vi "OE1022D_Read 1 parameter_mean.vi"(1 "数据转换":u8[](array[numeric]), 5 "Parameter 3":u16(ring) items=["AUX1", "AUX2", "AUX3", "AUX4"], 7 "Parameter 2":u16(ring) items=["X", "Y", "R", "Theta", "Frequency", "Noise", "Xh1", "Yh1", "Rh1", "Theta h1", "Xh2", "Yh2", "Rh2", "Theta h2"], 8 "错误输入（无错误）":errorcluster {"code" format="%f"}, 9 "Parameter":u16(ring) items=["X", "Y", "R", "Theta", "Frequency", "Noise", "Xh1", "Yh1", "Rh1", "Theta h1", "Xh2", "Yh2", "Rh2", "Theta h2"], 10 "Channel (0: A)":u16(ring) items=["Channel A", "Channel B", "ADC"], 11 "VISA resource name":refnum<visa-resource-name>) -> (0 "error out":errorcluster, 2 "Measurement":dbl format="%.3p", 3 "VISA resource name out":refnum<visa-resource-name>)   [LabVIEW 2022 SP3]
uses:
  <vilib>/Analysis/NI_AALBase.lvlib
panel:
  out "Measurement STD":dbl format="%#_13g"
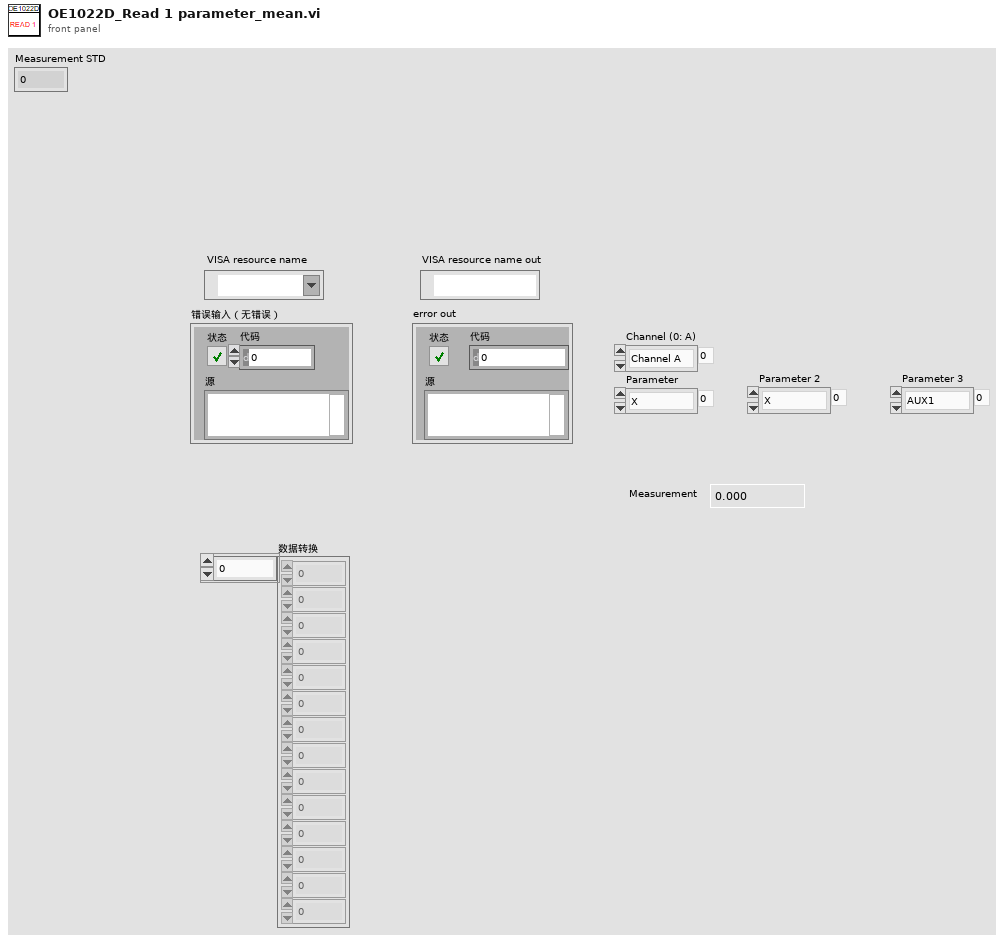
[diagram p1: front panel]
types:
  T1 = cluster{"AD1":dbl[], "AD2":dbl[], "AD3":dbl[], "AD4":dbl[]}
  T2 = cluster{"XA":dbl[], "YA":dbl[], "FrequencyA":dbl[], "NoiseA":dbl[], "Xh1A":dbl[], "Yh1A":dbl[], "Xh2A":dbl[], "Yh2A":dbl[]}
  T3 = cluster{"XB":dbl[], "YB":dbl[], "FrequencyB":dbl[], "NoiseB":dbl[], "Xh1B":dbl[], "Yh1B":dbl[], "Xh2B":dbl[], "Yh2B":dbl[], "Xh2B":dbl[]}
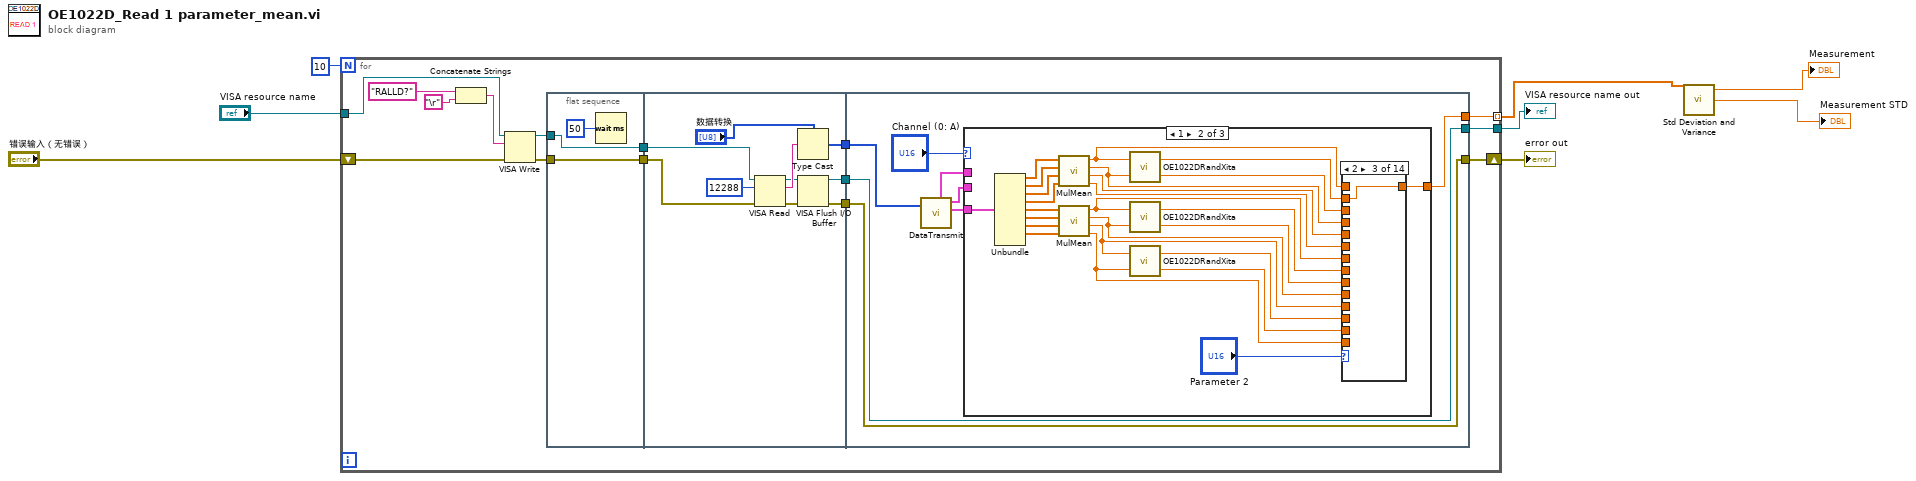
[diagram p0: block diagram]
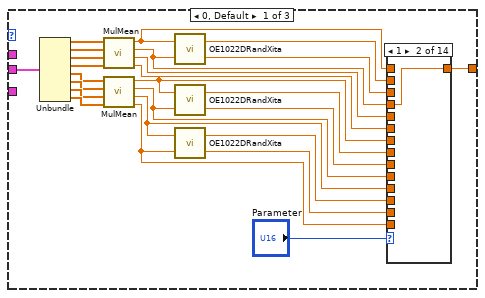
[diagram p2: hidden frame]
diagram:
  n1 = for {
    N: 10 -> [_]
    tunnel: [w13] -> w8
    shift-right: [w12] -> w7
    shift-left: "错误输入（无错误）" -> [w9]
    tunnel: [w11] -> w3 mode=indexing
    tunnel: "VISA resource name" -> [w10]
    n2 = Concatenate Strings("RALLD?" ("命令输入"), "\r") -> (w17:string)
    n3 = VISA Write(VISA resource name=w10, write buffer=w17, error in (no error)=w9) -> (VISA resource name out=w15:refnum<visa-resource-name>, error out=w14:errorcluster)  [unwired: 1 out]
    n4 = flat-sequence {
      tunnel: w15 -> [w24]
      tunnel: w14 -> [w25]
      tunnel: [w25] -> w23
      tunnel: [w24] -> w22
      tunnel: w23 -> [w28]
      tunnel: w22 -> [w27]
      tunnel: [w31] -> w21
      tunnel: [w30] -> w20
      tunnel: [w29] -> w19
      tunnel: w21 -> [w41]
      tunnel: w20 -> [w43]
      tunnel: w19 -> [w42]
      tunnel: [w43] -> w12
      tunnel: [w42] -> w13
      tunnel: [w37] -> w11
      frame #0 {
        n5 = Wait (ms)(milliseconds to wait=u32 50 ("等待时间（毫秒）")) -> ()  [unwired: 1 out]
      }
      frame #1 {
        n6 = VISA Read(VISA resource name=w27, byte count=12288, error in (no error)=w28) -> (VISA resource name out=w33:refnum<visa-resource-name>, read buffer=w35:string, error out=w34:errorcluster)  [unwired: 1 out]
        n7 = Type Cast(type="数据转换", x=w35) -> (*(type *) &x=w31:u8[])
        n8 = VISA Flush I/O Buffer(VISA resource name=w33, error in (no error)=w34) -> (VISA resource name out=w29:refnum<visa-resource-name>, error out=w30:errorcluster)  [unwired: 1 in]
      }
      frame #2 {
        n9 = call "DataTransmit.vi"("数据输入"=w41) -> ("输出簇ADC"=w40:T1, "输出簇A"=w39:T2, "输出簇B"=w38:T3)  [unwired: 2 in, 2 out]
        n10 = case shown="1" "Channel (0: A)" {
          tunnel: w40 -> [_ _ w129]
          tunnel: w39 -> [w60 _ _]
          tunnel: w38 -> [_ w84 _]
          tunnel: [w55 w85 w123] -> w37
          frame 0, Default {
            n11 = Unbundle(w60) -> ("XA"=w61:dbl[], "YA"=w62:dbl[], "FrequencyA"=w63:dbl[], "NoiseA"=w64:dbl[], "Xh1A"=w65:dbl[], "Yh1A"=w66:dbl[], "Xh2A"=w67:dbl[], "Yh2A"=w68:dbl[])
            n12 = call "MulMean.vi"("IN 4"=w64, "IN 3"=w63, "IN 2"=w62, "IN 1"=w61) -> ("mean 4"=w49:dbl, "mean 3"=w50:dbl, "mean 2"=w58:dbl, "mean 1"=w59:dbl)  [unwired: 4 in]
            n13 = call "MulMean.vi"("IN 4"=w68, "IN 3"=w67, "IN 2"=w66, "IN 1"=w65) -> ("mean 4"=w47:dbl, "mean 3"=w48:dbl, "mean 2"=w53:dbl, "mean 1"=w54:dbl)  [unwired: 4 in]
            n14 = call "OE1022DRandXita.vi"("Y"=w58, "X"=w59) -> ("θ (°)"=w56:dbl, "R"=w57:dbl)
            n15 = call "OE1022DRandXita.vi"("Y"=w53, "X"=w54) -> ("θ (°)"=w51:dbl, "R"=w52:dbl)
            n16 = call "OE1022DRandXita.vi"("Y"=w47, "X"=w48) -> ("θ (°)"=w45:dbl, "R"=w46:dbl)
            n17 = case shown="1" "Parameter" {
              tunnel: w59 -> [w70 _ _ _ _ _ _ _ _ _ _ _ _ _]
              tunnel: w58 -> [_ w71 _ _ _ _ _ _ _ _ _ _ _ _]
              tunnel: w57 -> [_ _ w72 _ _ _ _ _ _ _ _ _ _ _]
              tunnel: w56 -> [_ _ _ w73 _ _ _ _ _ _ _ _ _ _]
              tunnel: [w70 w71 w72 w73 w74 w75 w76 w77 w78 w79 w80 w81 w82 w83] -> w55
              tunnel: w54 -> [_ _ _ _ _ _ w76 _ _ _ _ _ _ _]
              tunnel: w53 -> [_ _ _ _ _ _ _ w77 _ _ _ _ _ _]
              tunnel: w52 -> [_ _ _ _ _ _ _ _ w78 _ _ _ _ _]
              tunnel: w51 -> [_ _ _ _ _ _ _ _ _ w79 _ _ _ _]
              tunnel: w50 -> [_ _ _ _ w74 _ _ _ _ _ _ _ _ _]
              tunnel: w49 -> [_ _ _ _ _ w75 _ _ _ _ _ _ _ _]
              tunnel: w48 -> [_ _ _ _ _ _ _ _ _ _ w80 _ _ _]
              tunnel: w47 -> [_ _ _ _ _ _ _ _ _ _ _ w81 _ _]
              tunnel: w46 -> [_ _ _ _ _ _ _ _ _ _ _ _ w82 _]
              tunnel: w45 -> [_ _ _ _ _ _ _ _ _ _ _ _ _ w83]
              frame 0, Default {
              }
              frame 1 {
              }
              frame 2 {
              }
              frame 3 {
              }
              frame 4 {
              }
              frame 5 {
              }
              frame 6 {
              }
              frame 7 {
              }
              frame 8 {
              }
              frame 9 {
              }
              frame 10 {
              }
              frame 11 {
              }
              frame 12 {
              }
              frame 13 {
              }
            }
          }
          frame 1 {
            n18 = Unbundle(w84) -> ("XB"=w94:dbl[], "YB"=w93:dbl[], "FrequencyB"=w92:dbl[], "NoiseB"=w91:dbl[], "Xh1B"=w90:dbl[], "Yh1B"=w89:dbl[], "Xh2B"=w88:dbl[], "Yh2B"=w87:dbl[])  [unwired: 1 out]
            n19 = call "MulMean.vi"("IN 4"=w91, "IN 3"=w92, "IN 2"=w93, "IN 1"=w94) -> ("mean 4"=w104:dbl, "mean 3"=w103:dbl, "mean 2"=w96:dbl, "mean 1"=w95:dbl)  [unwired: 4 in]
            n20 = call "MulMean.vi"("IN 4"=w87, "IN 3"=w88, "IN 2"=w89, "IN 1"=w90) -> ("mean 4"=w106:dbl, "mean 3"=w105:dbl, "mean 2"=w100:dbl, "mean 1"=w99:dbl)  [unwired: 4 in]
            n21 = call "OE1022DRandXita.vi"("Y"=w96, "X"=w95) -> ("θ (°)"=w98:dbl, "R"=w97:dbl)
            n22 = call "OE1022DRandXita.vi"("Y"=w100, "X"=w99) -> ("θ (°)"=w102:dbl, "R"=w101:dbl)
            n23 = call "OE1022DRandXita.vi"("Y"=w106, "X"=w105) -> ("θ (°)"=w108:dbl, "R"=w107:dbl)
            n24 = case shown="2" "Parameter 2" {
              tunnel: w95 -> [w109 _ _ _ _ _ _ _ _ _ _ _ _ _]
              tunnel: w96 -> [_ w110 _ _ _ _ _ _ _ _ _ _ _ _]
              tunnel: w97 -> [_ _ w111 _ _ _ _ _ _ _ _ _ _ _]
              tunnel: w98 -> [_ _ _ w112 _ _ _ _ _ _ _ _ _ _]
              tunnel: [w109 w110 w111 w112 w113 w114 w115 w116 w117 w118 w119 w120 w121 w122] -> w85
              tunnel: w99 -> [_ _ _ _ _ _ w115 _ _ _ _ _ _ _]
              tunnel: w100 -> [_ _ _ _ _ _ _ w116 _ _ _ _ _ _]
              tunnel: w101 -> [_ _ _ _ _ _ _ _ w117 _ _ _ _ _]
              tunnel: w102 -> [_ _ _ _ _ _ _ _ _ w118 _ _ _ _]
              tunnel: w103 -> [_ _ _ _ w113 _ _ _ _ _ _ _ _ _]
              tunnel: w104 -> [_ _ _ _ _ w114 _ _ _ _ _ _ _ _]
              tunnel: w105 -> [_ _ _ _ _ _ _ _ _ _ w119 _ _ _]
              tunnel: w106 -> [_ _ _ _ _ _ _ _ _ _ _ w120 _ _]
              tunnel: w107 -> [_ _ _ _ _ _ _ _ _ _ _ _ w121 _]
              tunnel: w108 -> [_ _ _ _ _ _ _ _ _ _ _ _ _ w122]
              frame 0, Default {
              }
              frame 1 {
              }
              frame 2 {
              }
              frame 3 {
              }
              frame 4 {
              }
              frame 5 {
              }
              frame 6 {
              }
              frame 7 {
              }
              frame 8 {
              }
              frame 9 {
              }
              frame 10 {
              }
              frame 11 {
              }
              frame 12 {
              }
              frame 13 {
              }
            }
          }
          frame 2 {
            n25 = Unbundle By Name(w129) -> ("AD1"=w133:dbl[], "AD2"=w132:dbl[], "AD3"=w131:dbl[], "AD4"=w130:dbl[])
            n26 = call "MulMean.vi"("IN 4"=w130, "IN 3"=w131, "IN 2"=w132, "IN 1"=w133) -> ("mean 4"=w124:dbl, "mean 3"=w125:dbl, "mean 2"=w126:dbl, "mean 1"=w127:dbl)  [unwired: 4 in]
            n27 = case shown="0, Default" "Parameter 3" {
              tunnel: w127 -> [w134 _ _ _]
              tunnel: w126 -> [_ w135 _ _]
              tunnel: w125 -> [_ _ w136 _]
              tunnel: w124 -> [_ _ _ w137]
              tunnel: [w134 w135 w136 w137] -> w123
              frame 0, Default {
              }
              frame 1 {
              }
              frame 2 {
              }
              frame 3 {
              }
            }
          }
        }
      }
    }
  }
  "VISA resource name out" <- w8
  "error out" <- w7
  n28 = call <vilib>:"Std Deviation and Variance.vi"("X"=w3) -> ("mean"=→"Measurement":dbl, "standard deviation"=→"Measurement STD":dbl)  [unwired: 1 in, 1 out]
